vi "Get Is Taps Supported.vi"(8 "error in (no error)":errorcluster, 10 "Taps":i32(ring) items=["SingleTap", "DualTap", "QuadTap"], 11 "TLCamera reference":refnum<k24>) -> (0 "error out":errorcluster, 2 "Is Taps Supported":bool, 3 "TLCamera reference out":refnum<k24>)   [LabVIEW 2020]
uses:
  C:/GEECS/Developers Version/builds/Device builds/ThorlabsCsCamera/Thorlabs.TSI.TLCameraInterfaces.dll
  Thorlabs.TSI.TLCameraInterfaces.dll
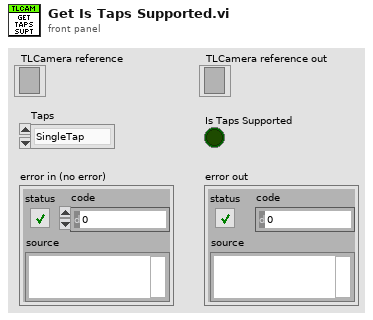
[diagram p1: front panel]
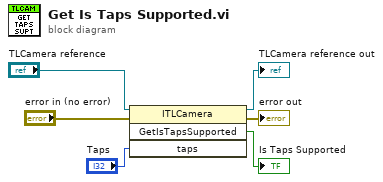
[diagram p0: block diagram]
diagram:
  n1 = invoke class="ITLCamera" method="GetIsTapsSupported"(reference="TLCamera reference", error in="error in (no error)", "taps"="Taps") -> (reference out=→"TLCamera reference out":refnum<k24>, error out=→"error out":errorcluster, "GetIsTapsSupported"=→"Is Taps Supported":bool)  [unwired: 1 in, 1 out]
